vi "Main.vi"() -> ()   [LabVIEW 2013]
panel:
  in  "stop":bool
  in  "VISA resource name":refnum<visa-resource-name>="COM6"
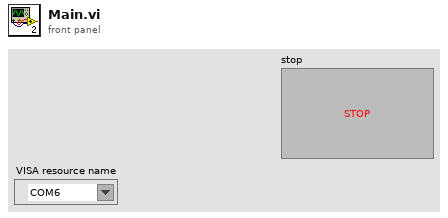
[diagram p1: front panel]
types:
  T1 = cluster{"PCStatusCMD":refnum<notifier>, "StarboardMotorCMD":refnum<notifier>, "PortMotorCMD":refnum<notifier>, "RightRudderCMD":refnum<notifier>, "LeftRudderCMD":refnum<notifier>, "PanCameraCMD":refnum<notifier>, "IR0CMD":refnum<notifier>, "Stop":refnum<notifier>}
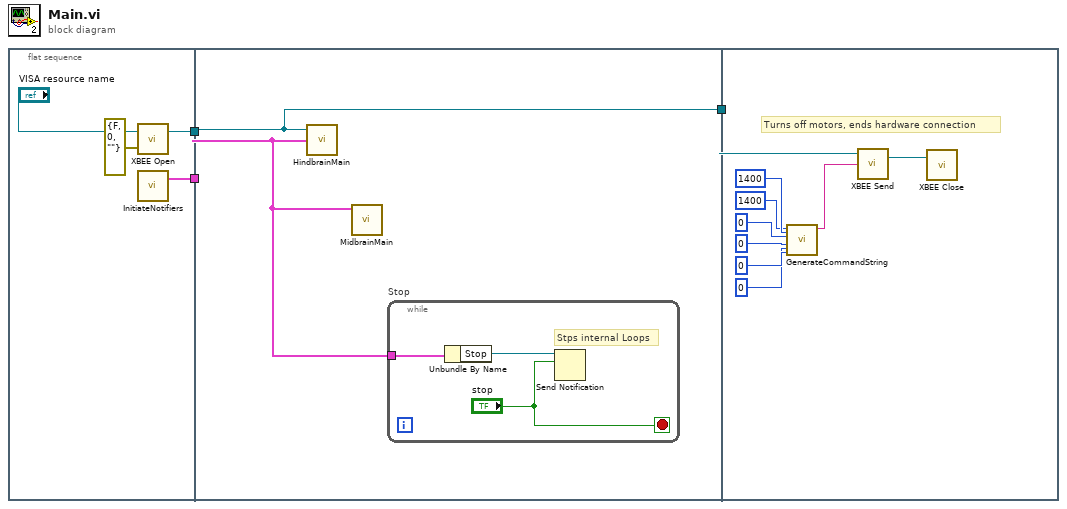
[diagram p0: block diagram]
diagram:
  n1 = flat-sequence {
    tunnel: [w5] -> w3
    tunnel: [w4] -> w2
    tunnel: w3 -> [w8]
    tunnel: w2 -> [w9]
    tunnel: [w8] -> w1
    tunnel: w1 -> [w21]
    frame #0 {
      n2 = call "XBEE Open.vi"("error in"=errorcluster {"status"=FALSE, "code"=0, "source"=""}, "VISA resource name"="VISA resource name") -> ("VISA resource name out"=w5:refnum<visa-resource-name>)  [unwired: 1 out]
      n3 = call "InitiateNotifiers.vi"() -> ("Notifiers"=w4:T1)  [unwired: 3 in]
    }
    frame #1 {
      n4 = call "HindbrainMain.vi"("Notifiers"=w9, "XBEE Refference"=w8) -> ()  [unwired: 6 in, 1 out]
      n5 = call "MidbrainMain.vi"("Notifiers"=w9) -> ()  [unwired: 11 in]
      n6 = while "Stop" {
        tunnel: w9 -> [w11]
        stop <- "stop" stop-if-true
        # "Stps internal Loops"
        n7 = Unbundle By Name(w11) -> ("Stop"=w10:refnum<notifier>)
        n8 = Send Notification(notification="stop", notifier=w10) -> ()  [unwired: 1 in, 2 out]
      }
    }
    frame #2 {
      # "Turns off motors, ends hardware connection"
      n9 = call "GenerateCommandString.vi"("Right Rubber"=0, "Port\nMotor"=1400 ("Port\nMotor"), "Pan Camera"=0, "Left Rudder"=0, "Starboard\nMotor"=0 ("Starboard\nMotor"), "PC Status"=1400) -> ("CommandString"=w19:string)  [unwired: 5 in]
      n10 = call "XBEE Send.vi"("String"=w19, "VISA resource name"=w21) -> ("VISA resource name out"=w20:refnum<visa-resource-name>)  [unwired: 1 in, 2 out]
      n11 = call "XBEE Close.vi"("VISA resource name"=w20) -> ()  [unwired: 1 in]
    }
  }
